vi "Import File - Common Block XML.vi"(6 "Root Node":refnum<k24>, 8 "error in (no error)":errorcluster) -> (0 "error out":errorcluster, 4 "Common":T1)   [LabVIEW 2016, in "UDP-Custom-Device System Explorer.lvlib"]
uses:
  UDP-Custom-Device System Explorer.lvlib
  System.Xml
  <vilib>/NI Veristand/Custom Device API/Custom Device Item Info.ctl
  <vilib>/NI VeriStand/Custom Device API/Custom Device API.lvlib
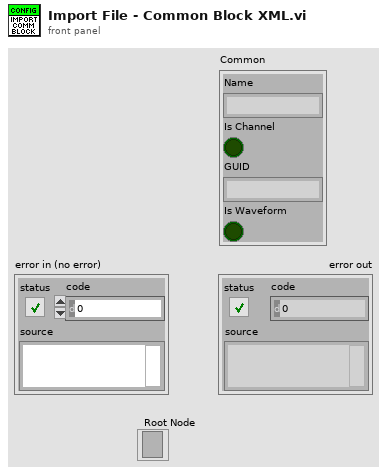
[diagram p1: front panel]
types:
  T1 = typedef "Custom Device API.lvlib/Custom Device Item Info.ctl" = cluster{"Name":string, "Is Channel":bool, "GUID":string, "Is Waveform":bool}
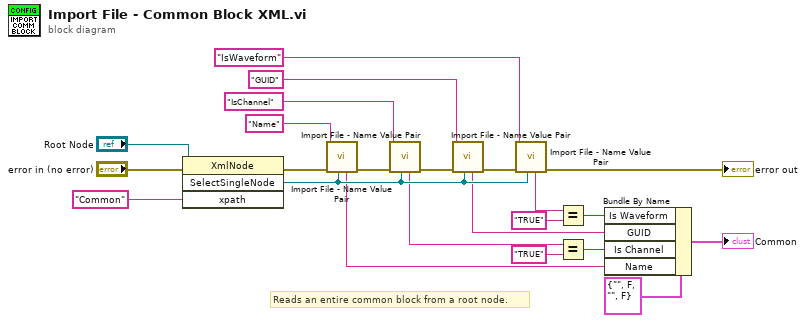
[diagram p0: block diagram]
diagram:
  # "Reads an entire common block from a root node."
  n1 = invoke class="XmlNode" method="SelectSingleNode"(reference="Root Node", error in="error in (no error)", "xpath"="Common") -> (error out=w16:errorcluster, "SelectSingleNode"=w10:refnum<k24>)  [unwired: 1 in, 2 out]
  n2 = call "Import File - Name Value Pair.vi"("Root Node"=w10, "error in (no error)"=w16, "Node Name"="Name" ("xpath")) -> ("error out"=w19:errorcluster, "Value"=w9:string)  [unwired: 7 in]
  n3 = call "Import File - Name Value Pair.vi"("Root Node"=w10, "error in (no error)"=w19, "Node Name"="IsChannel" ("xpath")) -> ("error out"=w18:errorcluster, "Value"=w3:string)  [unwired: 7 in]
  n4 = call "Import File - Name Value Pair.vi"("Root Node"=w10, "error in (no error)"=w18, "Node Name"="GUID" ("xpath")) -> ("error out"=w17:errorcluster, "Value"=w5:string)  [unwired: 7 in]
  n5 = call "Import File - Name Value Pair.vi"("Root Node"=w10, "error in (no error)"=w17, "Node Name"="IsWaveform" ("xpath")) -> ("error out"=→"error out":errorcluster, "Value"=w7:string)  [unwired: 7 in]
  n6 = Equal?(x=w7, y="TRUE") -> (x = y?=w1:bool)
  n7 = Equal?(x=w3, y="TRUE") -> (x = y?=w2:bool)
  n8 = Bundle By Name(cluster=T1 {"Name"="", "Is Channel"=FALSE, "GUID"="", "Is Waveform"=FALSE} ("Common"), "Is Waveform"=w1, "GUID"=w5, "Is Channel"=w2, "Name"=w9) -> (→"Common":T1)
